vi "LinearToDBFS.vi"(1 "Linear":dbl) -> (0 "dBFS":dbl)   [LabVIEW 2016]
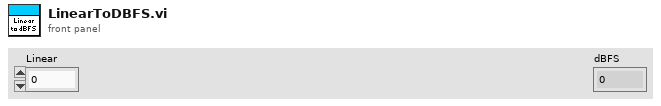
[diagram p1: front panel]
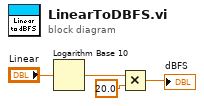
[diagram p0: block diagram]
diagram:
  n1 = Logarithm Base 10(1:"Linear") -> (0:w3:dbl)
  n2 = Multiply(x=w3, y=20.0) -> (x*y=→"dBFS":dbl)
